vi "Reserve Transfer_wrapper.vi"(7 "Description":string="Reserve", 8 "Command Info 2":T1, 11 "Command Name":string) -> (0 "Command Info":T1)   [LabVIEW 2025]
uses:
  <vilib>/Rock Robotics/WPI/Framework/Command Status Info.ctl
  <vilib>/Rock Robotics/WPI/Framework/Completion Status.ctl
  <vilib>/Rock Robotics/WPI/Framework/Completion Notifier.ctl
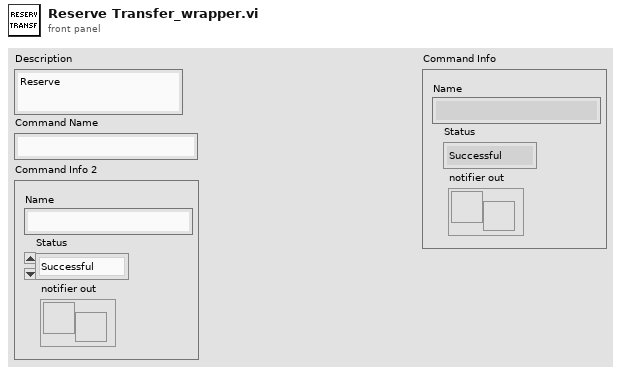
[diagram p1: front panel]
types:
  T1 = typedef "Command Status Info.ctl" = cluster{"Name":string, "Status":T2, "notifier out":T3}
  T2 = typedef "Completion Status.ctl" = enum16{"Successful", "Aborted", "Incomplete"}
  T3 = typedef "Completion Notifier.ctl" = refnum<notifier>
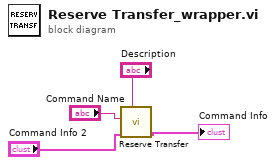
[diagram p0: block diagram]
diagram:
  n1 = call "Reserve Transfer.vi"("Description"="Description", "Command Info"="Command Info 2", "Command Name"="Command Name") -> ("Command Info"=→"Command Info":T1)  [unwired: 8 in]
